vi "Create.vi"(7 "user interface type":T1, 8 "error in (no error)":errorcluster, 11 "Components":refnum<class "Component.lvclass">[](array[class])) -> (0 "error out":errorcluster, 3 "Component Settings Editor":refnum<class "Component Settings Editor.lvclass">)   [LabVIEW 2017, in "DSF Core.lvlib" / "Component Settings Editor.lvclass"]
uses:
  Component Settings Editor.lvclass
  Component/Component.lvclass
  Component User Interface/UI Type.ctl
  Component Settings Editor.lvclass/Component Settings Editor.ctl
  Component User Interface/Component User Interfaces.lvclass
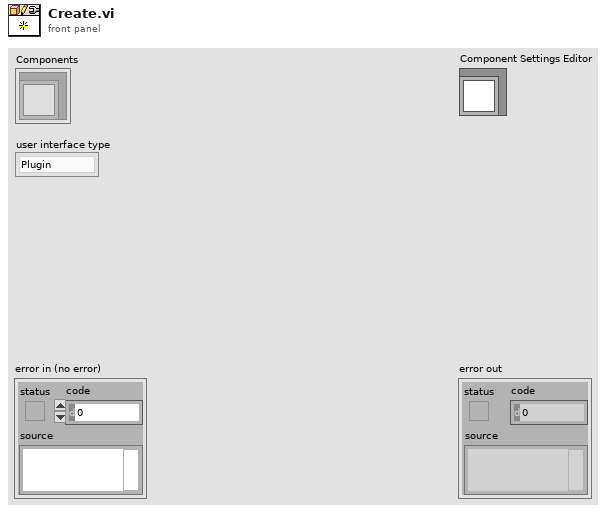
[diagram p1: front panel]
types:
  T1 = typedef "DSF Core.lvlib/Component User Interfaces.lvclass/UI Type.ctl" = enum16{"Plugin", "Thread", "Rx Group", "Tx Group", "Rx Transfer", "Tx Transfer", "Rx Channel", "Tx Channel"}
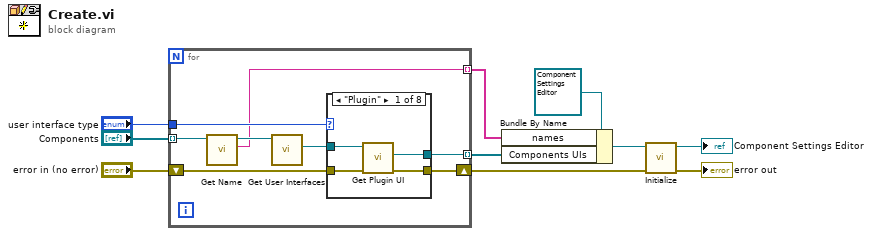
[diagram p0: block diagram]
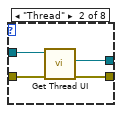
[diagram p2: hidden frame]
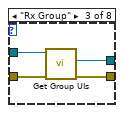
[diagram p3: hidden frame]
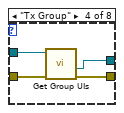
[diagram p4: hidden frame]
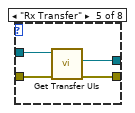
[diagram p5: hidden frame]
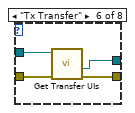
[diagram p6: hidden frame]
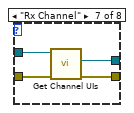
[diagram p7: hidden frame]
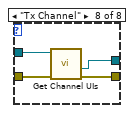
[diagram p8: hidden frame]
diagram:
  n1 = for {
    tunnel: "Components" -> [w18] mode=indexing
    tunnel: [w13] -> w8 mode=indexing
    tunnel: [w11] -> w5 mode=indexing
    tunnel: "user interface type" -> [w15]
    shift-right: [w12] -> w4
    shift-left: "error in (no error)" -> [w14]
    n2 = call "Get Name.vi"("Component in"=w18) -> ("name"=w13:string, "Component out"=w17:refnum<class "Component.lvclass">)  [unwired: 9 in]
    n3 = call "Get User Interfaces.vi"("Component in"=w17) -> ("User Interfaces"=w16:refnum<class "Component User Interfaces.lvclass">)  [unwired: 9 in, 1 out]
    n4 = case shown="\"Plugin\"" w15 {
      tunnel: [w22 w26 w30 w33 w38 w41 w43 w47] -> w11
      tunnel: w16 -> [w21 w25 w29 w34 w37 w42 w46 w50]
      tunnel: [w20 w23 w27 w31 w35 w39 w44 w48] -> w12
      tunnel: w14 -> [w19 w24 w28 w32 w36 w40 w45 w49]
      frame "Plugin" {
        n5 = call-dynamic "Get Plugin UI.vi"("error in (no error)"=w19, "Component UI in"=w21) -> ("error out"=w20:errorcluster, "Plugin Settings UI"=w22:refnum<class "User Interface.lvclass">)  [unwired: 7 in, 1 out]
      }
      frame "Thread" {
        n6 = call-dynamic "Get Thread UI.vi"("error in (no error)"=w24, "Component UI in"=w25) -> ("error out"=w23:errorcluster, "Thread Settings UI"=w26:refnum<class "User Interface.lvclass">)  [unwired: 7 in, 1 out]
      }
      frame "Rx Group" {
        n7 = call-dynamic "Get Group UIs.vi"("error in (no error)"=w28, "Component UI in"=w29) -> ("error out"=w27:errorcluster, "Rx Group UI"=w30:refnum<class "User Interface.lvclass">)  [unwired: 6 in, 2 out]
      }
      frame "Tx Group" {
        n8 = call-dynamic "Get Group UIs.vi"("error in (no error)"=w32, "Component UI in"=w34) -> ("error out"=w31:errorcluster, "Tx Group UI"=w33:refnum<class "User Interface.lvclass">)  [unwired: 6 in, 2 out]
      }
      frame "Rx Transfer" {
        n9 = call-dynamic "Get Transfer UIs.vi"("error in (no error)"=w36, "Component UI in"=w37) -> ("error out"=w35:errorcluster, "Rx Transfer UI"=w38:refnum<class "User Interface.lvclass">)  [unwired: 6 in, 2 out]
      }
      frame "Tx Transfer" {
        n10 = call-dynamic "Get Transfer UIs.vi"("error in (no error)"=w40, "Component UI in"=w42) -> ("error out"=w39:errorcluster, "Tx Transfer UI"=w41:refnum<class "User Interface.lvclass">)  [unwired: 6 in, 2 out]
      }
      frame "Rx Channel" {
        n11 = call-dynamic "Get Channel UIs.vi"("error in (no error)"=w45, "Component UI in"=w46) -> ("error out"=w44:errorcluster, "Rx Channel UI"=w43:refnum<class "User Interface.lvclass">)  [unwired: 6 in, 2 out]
      }
      frame "Tx Channel" {
        n12 = call-dynamic "Get Channel UIs.vi"("error in (no error)"=w49, "Component UI in"=w50) -> ("error out"=w48:errorcluster, "Tx Channel UI"=w47:refnum<class "User Interface.lvclass">)  [unwired: 6 in, 2 out]
      }
    }
  }
  n13 = Bundle By Name(cluster=refnum<class "Component Settings Editor.lvclass"> refnum ("Component Settings Editor in"), "names"=w8, "Components UIs"=w5) -> (w2:refnum<class "Component Settings Editor.lvclass">)
  n14 = call-dynamic "Initialize.vi"("error in (no error)"=w4, "Component Settings Editor in"=w2) -> ("error out"=→"error out":errorcluster, "Component Settings Editor out"=→"Component Settings Editor":refnum<class "Component Settings Editor.lvclass">)  [unwired: 8 in]
